vi "Avrg_minute_hour_day.vi"(0 "MCU addresses":T2="B", 5 "Data ID Nr":T1 items=["", "", "", "", "", "MCU ADRESS", "", "", "", "", "ACC X", "ACC Y", "ACC Z", "ACC LEN", "TIME HOURS", "TIME MINUTS", "TIME SECONDS", "ZIGBEE TEMP", "INSIDE TEMP", "OUTSIDE TEMP", "POT111", "PIR SENSOR", "LIGHT SENSOR", "", "", "DOOR STAUS_1", "DOOR STAUS_1", "", "", "", "Empty", "Empty", "Empty", "", "", "", "", "", "", "", "", "", "", "", "", "", "", "", "", "", "", "", "", "", "", "", "", "", "", "", "", "Empty"]) -> (4 "Average over a minute":dbl, 6 "Average over an hour":dbl, 8 "Average over a day":dbl, 10 "Max Value":dbl, 15 "Min Value":dbl)   [LabVIEW 2016]
uses:
  Typedef/MCU_addresses.ctl
  Typedef/Data_ID.ctl
  <vilib>/Utility/file.llb/Read Delimited Spreadsheet (DBL).vi
panel:
  out "nearest integer value 4":dbl
  out "nearest integer value 3":dbl
  out "size(s)":i32[](array[numeric])
  out "path":path
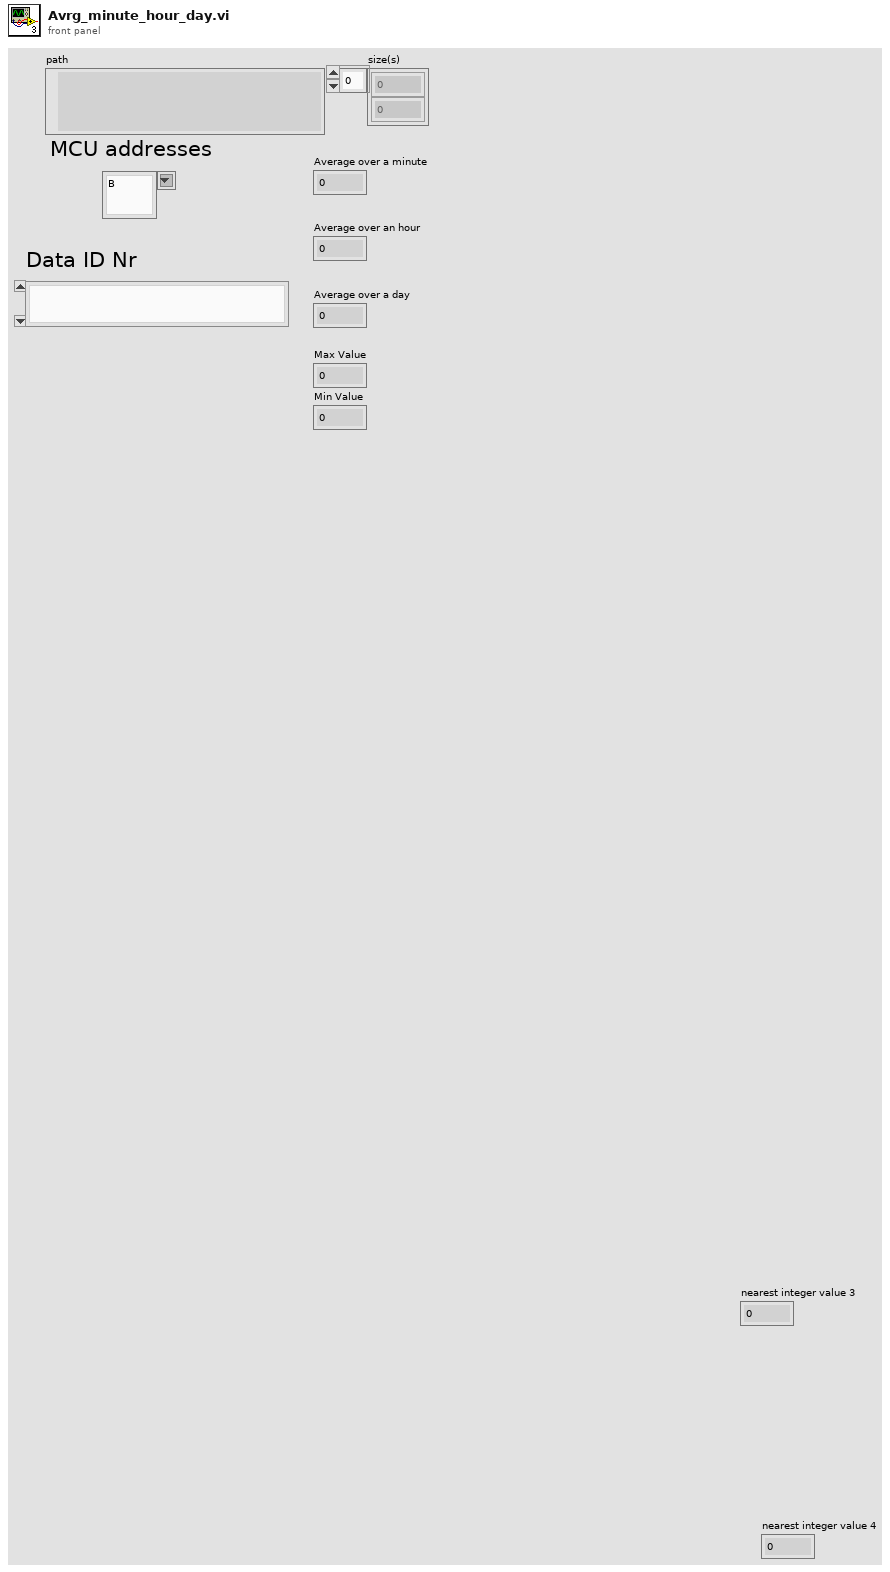
[diagram p1: front panel]
types:
  T1 = typedef "Data_ID.ctl" = u16
  T2 = typedef "MCU_addresses.ctl" = string
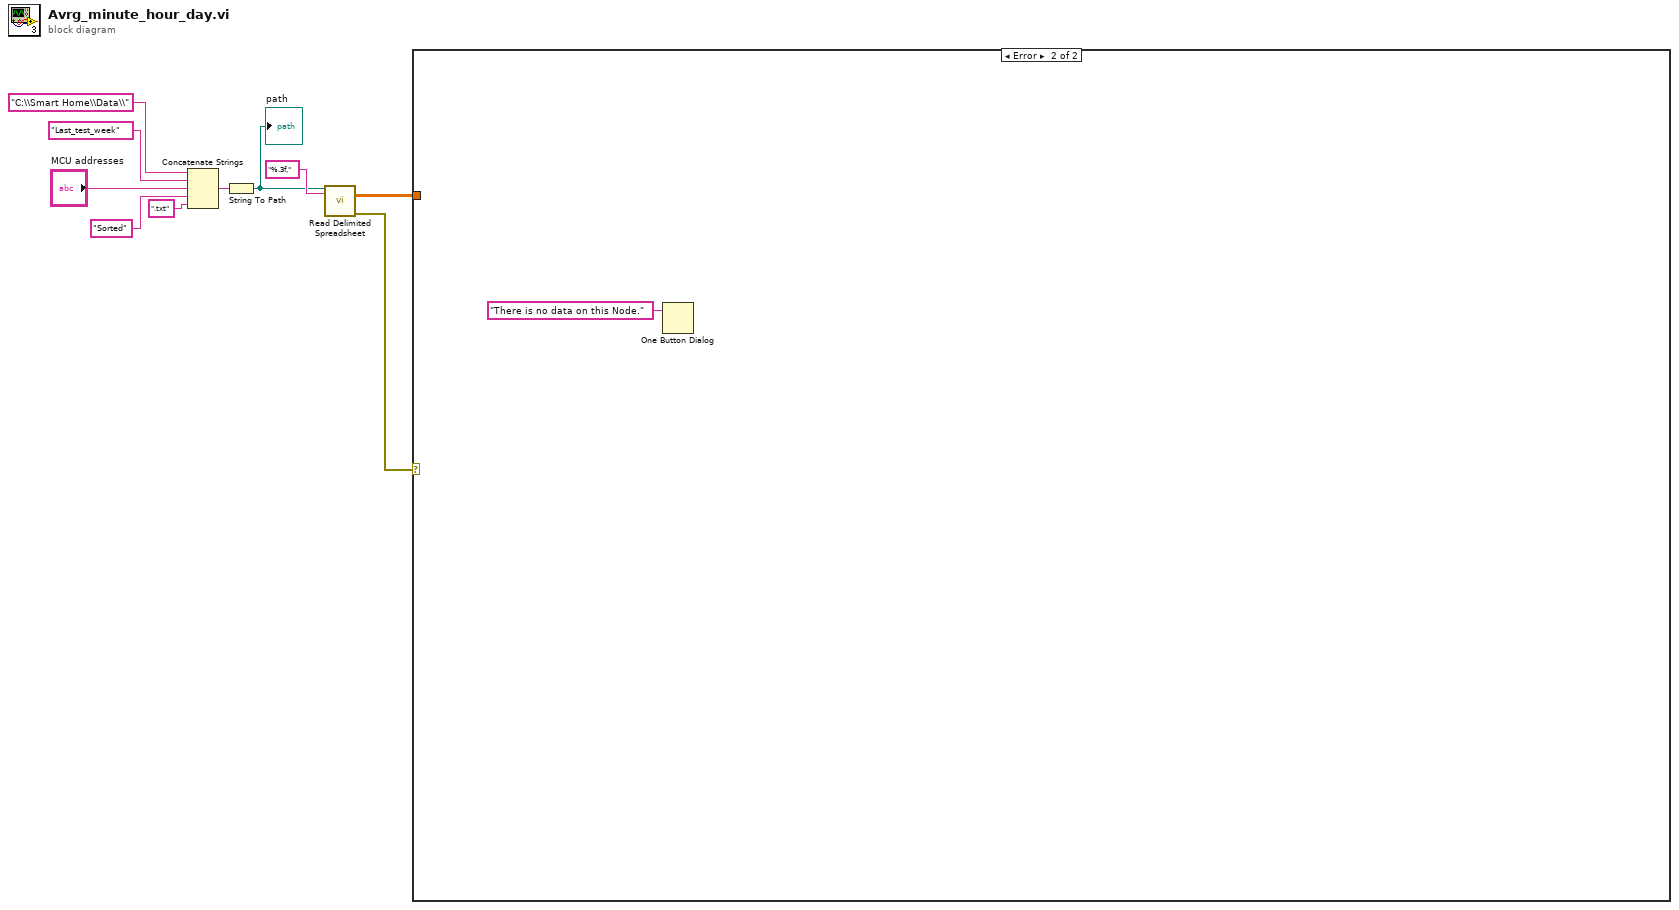
[diagram p0: block diagram]
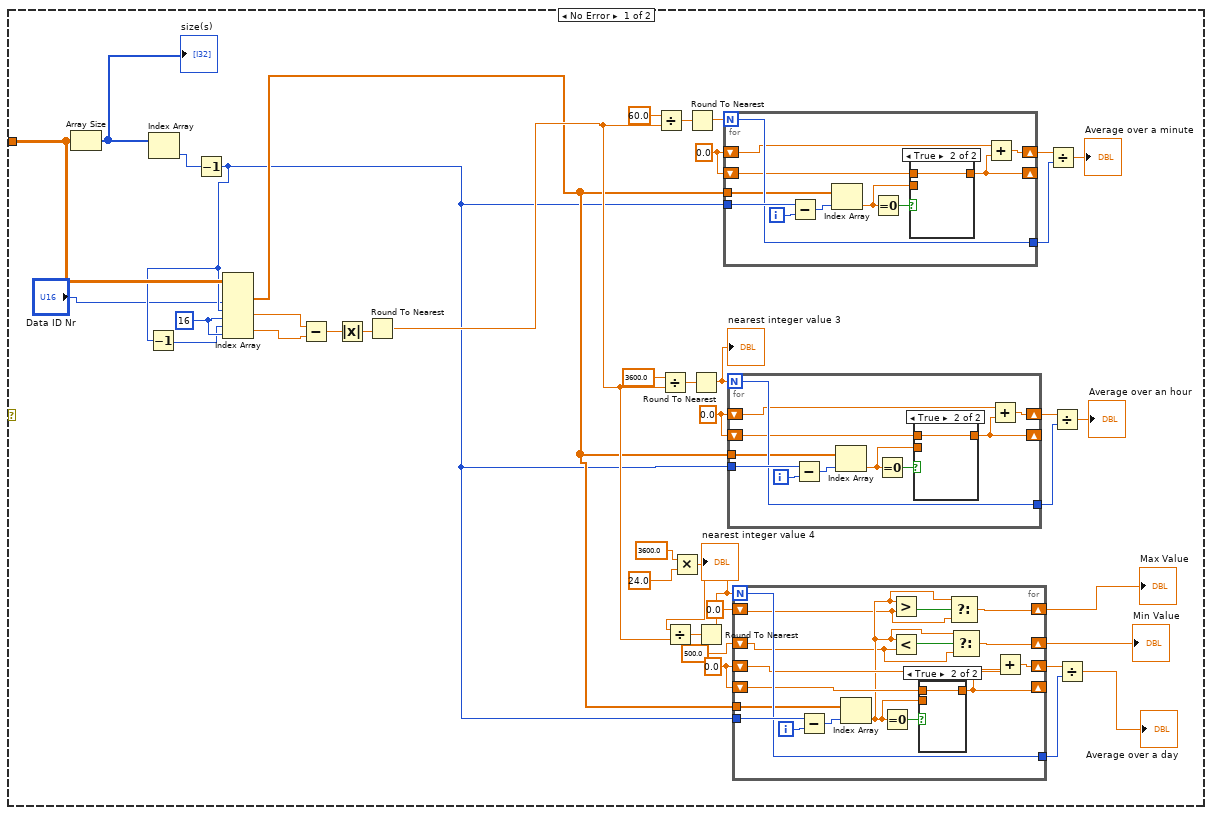
[diagram p2: hidden frame]
diagram:
  n1 = Concatenate Strings("C:\\Smart Home\\Data\\", "Last_test_week" ("String"), "MCU addresses", "Sorted" ("string"), ".txt") -> (w10:string)
  n2 = String To Path(string=w10) -> (path=w3:path)
  "path" <- w3
  n3 = call-poly <vilib>:"Read Delimited Spreadsheet.vi"("file path (dialog if empty)"=w3, "format (%.3f)"="%.3f,") -> ("all rows"=w2:dbl[][], "error out"=w1:errorcluster)  [unwired: 8 in, 4 out]
  n4 = case shown="Error" w1 {
    tunnel: w2 -> [w50 _]
    frame No Error {
      w11 = 0.0 ("Numeric")
      w13 = 0.0 ("Numeric")
      w12 = 0.0 ("Numeric")
      w48 = 16 ("index (col)")
      n5 = Array Size(array=w50) -> (size(s)=w49:i32[])
      "size(s)" <- w49
      n6 = Index Array(array=w49) -> (element=w46:i32)  [unwired: 1 in]
      n7 = Decrement(x=w46) -> (x-1=w19:i32)
      n8 = Decrement(x=w19) -> (x-1=w47:i32)
      n9 = Index Array(array=w50, index (col) #1="Data ID Nr", index (row) #2=w19, index (col) #2=w48, index (row) #3=w47, index (col) #3=w48) -> (element #1=w20:dbl[], element #2=w45:dbl, element #3=w44:dbl)  [unwired: 1 in]
      n10 = Subtract(x=w45, y=w44) -> (x-y=w43:dbl)
      n11 = Absolute Value(x=w43) -> (abs(x)=w42:dbl)
      n12 = Round To Nearest(number=w42) -> (nearest integer value=w24:dbl)
      n13 = Divide(x=60.0, y=w24) -> (x/y=w38:dbl)
      n14 = Divide(x=3600.0, y=w24) -> (x/y=w32:dbl)
      n15 = Multiply(x=3600.0, y=24.0) -> (x*y=w21:dbl)
      n16 = Divide(x=w21, y=w24) -> (x/y=w26:dbl)
      n17 = Round To Nearest(number=w38) -> (nearest integer value=w37:dbl)
      n18 = Round To Nearest(number=w32) -> (nearest integer value=w31:dbl)
      "nearest integer value 3" <- w31
      n19 = Round To Nearest(number=w26) -> (nearest integer value=w25:dbl)
      "nearest integer value 4" <- w25
      n20 = for {
        N: w37 -> [w89]
        tunnel: w19 -> [w91]
        shift-right: [w90] -> w40
        shift-left: w12 -> [w86]
        tunnel: [w89] -> w41
        tunnel: w20 -> [w88]
        shift-right: [w84] -> _
        shift-left: w12 -> [w83]
        i -> [w92]
        n21 = Subtract(x=w91, y=w92) -> (x-y=w93:i32)
        n22 = Index Array(array=w88, index=w93) -> (element=w85:dbl)
        n23 = Equal To 0?(x=w85) -> (x = 0?=w87:bool)
        n24 = case shown="True" w87 {
          tunnel: [w94 w95] -> w84
          tunnel: w85 -> [w94 _]
          tunnel: w83 -> [_ w95]
          frame False {
          }
          frame True {
          }
        }
        n25 = Add(x=w86, y=w84) -> (x+y=w90:dbl)
      }
      n26 = for {
        N: w31 -> [w76]
        tunnel: w19 -> [w78]
        shift-right: [w77] -> w34
        shift-left: w13 -> [w73]
        tunnel: [w76] -> w35
        tunnel: w20 -> [w75]
        shift-right: [w71] -> _
        shift-left: w13 -> [w70]
        i -> [w79]
        n27 = Subtract(x=w78, y=w79) -> (x-y=w80:i32)
        n28 = Index Array(array=w75, index=w80) -> (element=w72:dbl)
        n29 = Equal To 0?(x=w72) -> (x = 0?=w74:bool)
        n30 = case shown="True" w74 {
          tunnel: [w81 w82] -> w71
          tunnel: w72 -> [w81 _]
          tunnel: w70 -> [_ w82]
          frame False {
          }
          frame True {
          }
        }
        n31 = Add(x=w73, y=w71) -> (x+y=w77:dbl)
      }
      n32 = for {
        N: w25 -> [w63]
        tunnel: w19 -> [w65]
        shift-right: [w64] -> w28
        shift-left: w11 -> [w57]
        tunnel: [w63] -> w29
        tunnel: w20 -> [w62]
        shift-right: [w56] -> _
        shift-left: w11 -> [w60]
        shift-right: [w54] -> w17
        shift-left: 0.0 ("Numeric") -> [w51]
        shift-right: [w55] -> w16
        shift-left: 500.0 ("Numeric") -> [w52]
        i -> [w66]
        n33 = Subtract(x=w65, y=w66) -> (x-y=w67:i32)
        n34 = Index Array(array=w62, index=w67) -> (element=w53:dbl)
        n35 = Equal To 0?(x=w53) -> (x = 0?=w61:bool)
        n36 = Greater?(x=w53, y=w51) -> (0:w59:bool)
        n37 = Less?(x=w53, y=w52) -> (x < y?=w58:bool)
        n38 = case shown="True" w61 {
          tunnel: [w68 w69] -> w56
          tunnel: w53 -> [w68 _]
          tunnel: w60 -> [_ w69]
          frame False {
          }
          frame True {
          }
        }
        n39 = Select(t=w53, s=w59, f=w51) -> (s? t:f=w54:dbl)
        n40 = Select(t=w53, s=w58, f=w52) -> (s? t:f=w55:dbl)
        n41 = Add(x=w57, y=w56) -> (x+y=w64:dbl)
      }
      "Max Value" <- w17
      "Min Value" <- w16
      n42 = Divide(x=w40, y=w41) -> (x/y=→"Average over a minute":dbl)
      n43 = Divide(x=w34, y=w35) -> (x/y=→"Average over an hour":dbl)
      n44 = Divide(x=w28, y=w29) -> (x/y=→"Average over a day":dbl)
    }
    frame Error {
      n45 = One Button Dialog(message="There is no data on this Node.") -> ()  [unwired: 1 in, 1 out]
    }
  }
